vi "Register Set Parse2.vi"(6 "Register Name":string, 8 "error in (no error)":errorcluster, 9 "Register value":u8 format="%.0x", 10 "Register Names":string[](array[string]), 11 "RegMap Data":T1[](array[typedef]) {"Base" format="%.0x"; "Item Count" format="%.0x"; "Value" format="%.0x"; "RegMap"."Mask" format="%.0x"; "Default" format="%.0x"; "Register" format="%.0x"}) -> (0 "error out":errorcluster, 3 "Register Value Array":u8[](array[numeric]))   [LabVIEW 2010]
doc: "This VI takes the register value and converts it into an array that represent the individual settings for that register. Each control group is assigned an array element with a[0] = least significant group (group containing the LSB)\n\nInputs:\nRegMap Data - (cluster[]) register map data for the device (scanned from file)\nRegister Names - (string[]) register names is same order as RegMap Data array (used for indexing/searching)\nRegister Name - (string) Name of the register that is being converted\nRegister Value - (int) value of register\nerror in - error input cluster\n\nOutputs:\nRegister Value Array - (int[]) contains values of each group within the register\nerror out - error output cluster"
uses:
  Scan RegMap/TYP_ADSxxxx Register.ctl
  Scan RegMap/TYP_RegMap Item.ctl
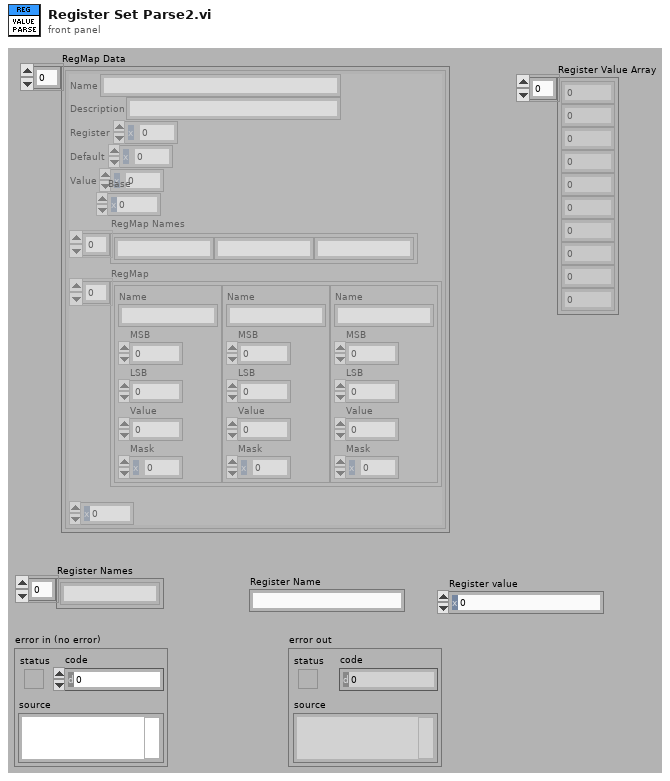
[diagram p1: front panel]
types:
  T1 = typedef "TYP_ADSxxxx Register.ctl" = cluster{"Name":string, "Description":string, "Register":u16, "Default":u16, "Value":u16, "Base":u16, "RegMap Names":string[], "RegMap":T2[], "Item Count":u8}
  T2 = typedef "TYP_RegMap Item.ctl" = cluster{"Name":string, "MSB":u16, "LSB":u16, "Value":u16, "Mask":u16}
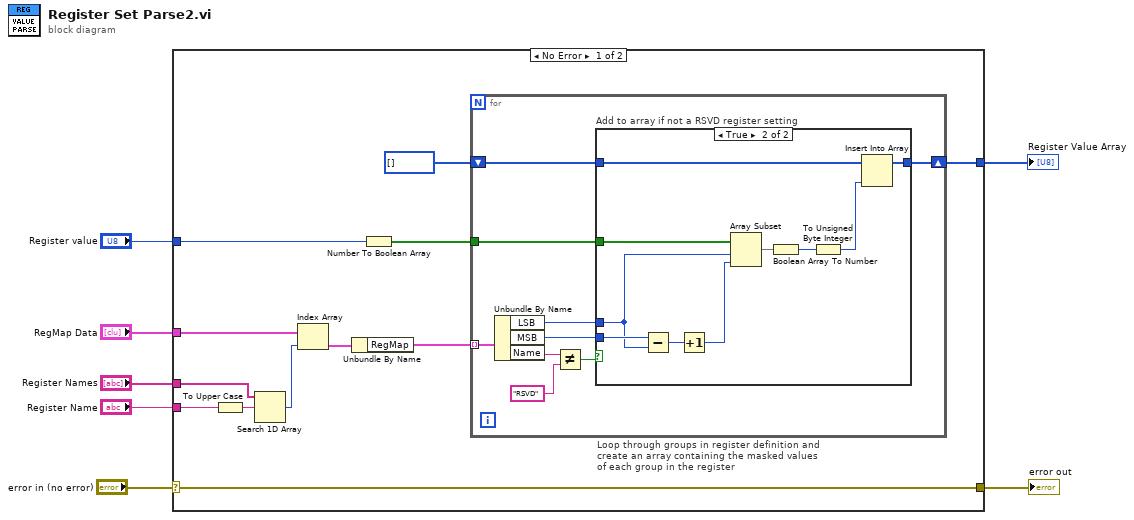
[diagram p0: block diagram]
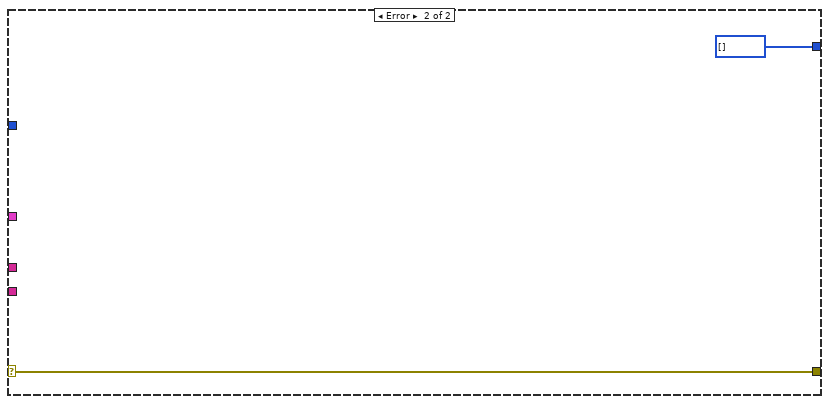
[diagram p3: hidden frame]
diagram:
  n1 = case shown="No Error" "error in (no error)" {
    selector: "error in (no error)" -> [w11 w41]
    tunnel: "Register value" -> [w19 _]
    tunnel: [w8 u8[] []] -> w6
    tunnel: "Register Name" -> [w17 _]
    tunnel: "Register Names" -> [w15 _]
    tunnel: "RegMap Data" -> [w14 _]
    tunnel: [w11 w41] -> w1
    frame No Error {
      n2 = To Upper Case(1:w17) -> (0:w16:string)
      n3 = Search 1D Array(1D array=w15, element=w16) -> (index of element=w18:i32)  [unwired: 1 out]
      n4 = Index Array(array=w14, index=w18) -> (element=w13:T1)
      n5 = Unbundle By Name(w13) -> ("RegMap"=w12:T2[])
      n6 = Number To Boolean Array(number=w19) -> (Boolean array=w10:bool[])
      n7 = for "Loop through groups in register definition and create an array containing the masked values\nof each group in the register" {
        tunnel: w10 -> [w28]
        tunnel: w12 -> [w26] mode=indexing
        shift-right: [w20] -> w8
        shift-left: u8[] [] -> [w21]
        n8 = Unbundle By Name(w26) -> ("LSB"=w25:u16, "MSB"=w27:u16, "Name"=w23:string)
        n9 = Not Equal?(x=w23, y="RSVD") -> (x != y?=w24:bool)
        n10 = case "Add to array if not a RSVD register setting" shown="True" w24 {
          tunnel: w28 -> [_ w39]
          tunnel: w27 -> [_ w38]
          tunnel: w25 -> [_ w35]
          tunnel: w21 -> [w29 w31]
          tunnel: [w29 w32] -> w20
          frame False {
          }
          frame True {
            n11 = Subtract(x=w38, y=w35) -> (x-y=w33:u16)
            n12 = Increment(x=w33) -> (x+1=w37:u16)
            n13 = Array Subset(array=w39, index=w35, length=w37) -> (w36:bool[])
            n14 = Boolean Array To Number(Boolean array=w36) -> (number=w34:u32)
            n15 = To Unsigned Byte Integer(number=w34) -> (unsigned 8bit integer=w30:u8)
            n16 = Insert Into Array(array=w31, new element=w30) -> (w32:u8[])  [unwired: 1 in]
          }
        }
      }
    }
    frame Error {
    }
  }
  "Register Value Array" <- w6
  "error out" <- w1
